vi "SETI_Host_Interface v2.vi"() -> ()   [LabVIEW 2012]
uses:
  SETI FPGA States.ctl
  <vilib>/rvi/Emulation/niFpgaSctlEmulationGetInTimedLoop.vi
  <vilib>/rvi/Emulation/niFpgaSctlEmulationGlobalWrite.vi
  <vilib>/rvi/interface/RandomDataEmulation/nirviRandomDataFPGAFIFO.vi
  <vilib>/rvi/interface/RandomDataEmulation/niFpgaRandomDataHandleErrors.vi
  <vilib>/rvi/DataTransferAndStorage/Container/XNode/niFpgaContainer.xnode
  <vilib>/rvi/interface/RandomDataEmulation/nirviRandomDataFpgaReadWriteTemplate.vi
panel:
  out "FPGA Loop Count":i32
  out "State":T1
  out "Total":u64
  out "Count":u64
  in  "Start":bool
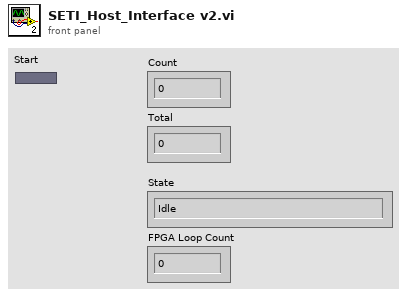
[diagram p1: front panel]
types:
  T1 = typedef "SETI FPGA States.ctl" = enum16{"Idle", "GetNumPoints", "GetChirpRate", "Process", "Stop"}
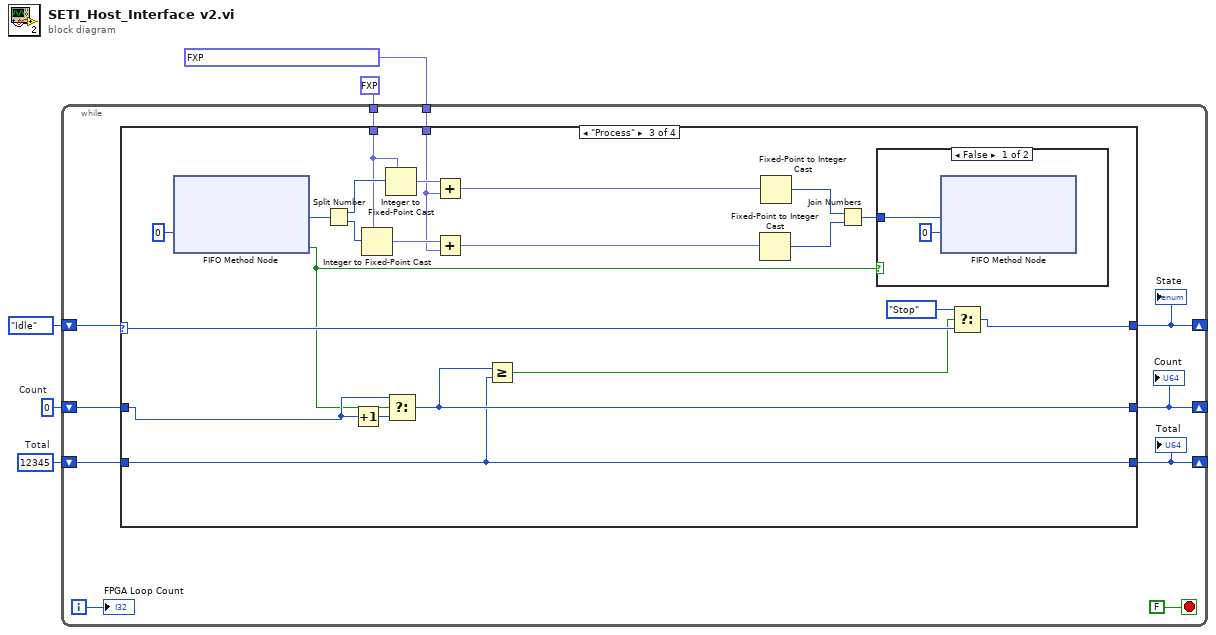
[diagram p0: block diagram]
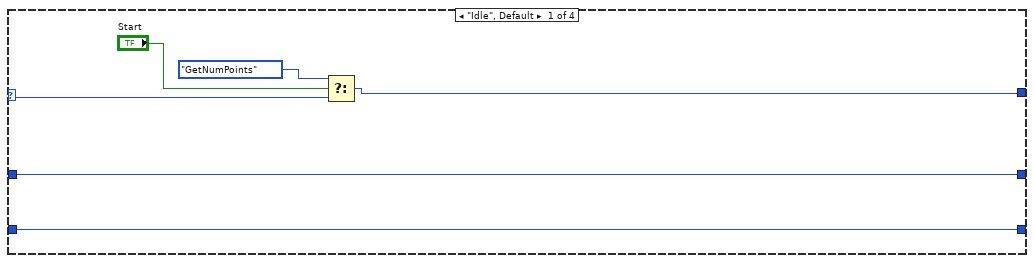
[diagram p2: hidden frame]
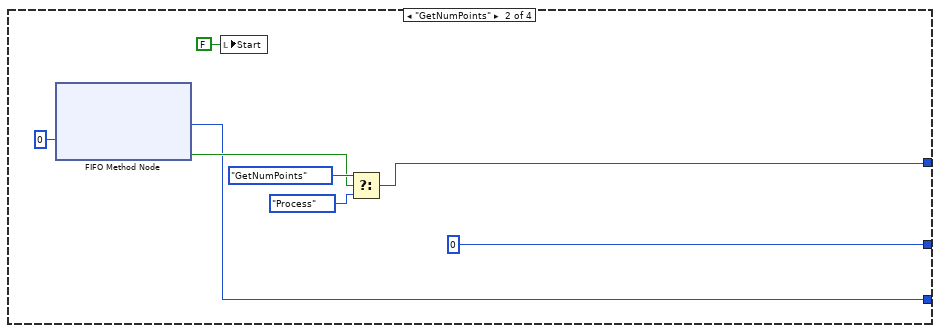
[diagram p3: hidden frame]
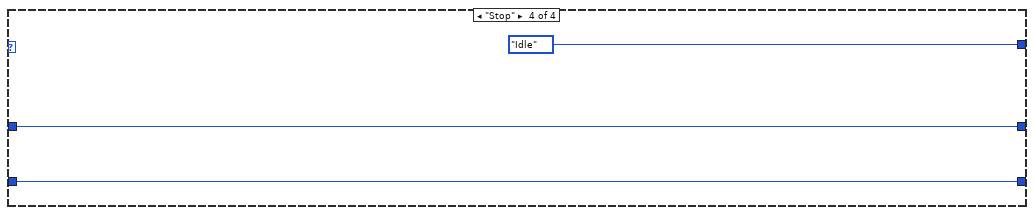
[diagram p5: hidden frame]
diagram:
  w3 = u64 12345  # Total
  w4 = u64 0  # Count
  n1 = while {
    shift-right: [w14] -> _
    shift-left: SETI_FPGA_States."Idle" -> [w15]
    shift-right: [w11] -> _
    shift-left: w4 -> [w12]
    shift-right: [w9] -> _
    shift-left: w3 -> [w10]
    tunnel: fxp<+/-,32,1> 0.0 ("real data in") -> [w7]
    tunnel: fxp<+/-,32,1> 0.2999999998137355 ("y") -> [w6]
    i -> [w8]
    stop <- FALSE stop-if-true
    n2 = case shown="\"Process\"" w15 {
      selector: w15 -> [w20 _ w49 _]
      tunnel: [w19 w23 w48 SETI_FPGA_States."Idle"] -> w14
      tunnel: w12 -> [w17 _ w50 w55]
      tunnel: [w17 u64 0 ("Timeout") w44 w55] -> w11
      tunnel: w10 -> [w16 _ w43 w54]
      tunnel: [w16 w22 w43 w54] -> w9
      tunnel: w7 -> [_ _ w35 _]
      tunnel: w6 -> [_ _ w32 _]
      frame "Idle", Default {
        n3 = Select(t=SETI_FPGA_States."GetNumPoints", s="Start", f=w20) -> (s? t:f=w19:T1)
      }
      frame "GetNumPoints" {
        n4 = xnode ("FIFO Method Node")("Timeout"=0) -> ("Element"=w22:u64, "Timed Out?"=w25:bool)  [unwired: 1 in, 1 out]
        n5 = local write "Start"(FALSE ("Start")) -> ()
        n6 = Select(t=SETI_FPGA_States."GetNumPoints", s=w25, f=SETI_FPGA_States."Process") -> (s? t:f=w23:T1)
      }
      frame "Process" {
        n7 = xnode ("FIFO Method Node")("Timeout"=0) -> ("Element"=w36:u64, "Timed Out?"=w42:bool)  [unwired: 1 in, 1 out]
        n8 = Split Number(x=w36) -> (hi(x)=w40:u32, lo(x)=w41:u32)
        n9 = Increment(x=w50) -> (x+1=w45:u64)
        n10 = Integer to Fixed-Point Cast(fixed-point type=w35, integer=w41) -> (fixed-point=w33:fxp<+/-,32,1>)
        n11 = Integer to Fixed-Point Cast(fixed-point type=w35, integer=w40) -> (fixed-point=w34:fxp<+/-,32,1>)
        n12 = Select(t=w50, s=w42, f=w45) -> (s? t:f=w44:u64)
        n13 = Add(x=w34, y=w32) -> (x+y=w30:fxp<+/-,33,2>)
        n14 = Add(x=w33, y=w32) -> (x+y=w31:fxp<+/-,33,2>)
        n15 = Greater Or Equal?(x=w44, y=w43) -> (x >= y?=w47:bool)
        n16 = Fixed-Point to Integer Cast(1:w31) -> (0:w38:i64)
        n17 = Fixed-Point to Integer Cast(1:w30) -> (0:w39:i64)
        n18 = Join Numbers(hi=w39, lo=w38) -> ((hi.lo)=w37:u64)
        n19 = case shown="False" w42 {
          tunnel: w37 -> [w53 _]
          frame False {
            n20 = xnode ("FIFO Method Node")("Element"=w53, "Timeout"=0) -> ()  [unwired: 1 in, 2 out]
          }
          frame True {
          }
        }
        n21 = Select(t=SETI_FPGA_States."Stop", s=w47, f=w49) -> (s? t:f=w48:T1)
      }
      frame "Stop" {
      }
    }
    "Count" <- w11
    "Total" <- w9
    "State" <- w14
    "FPGA Loop Count" <- w8
  }
